vi "Connect.vi"(8 "error in (no error)":errorcluster, 10 "BaudRate":u32, 11 "VisaResource":string) -> (0 "error out":errorcluster, 3 "T560Session out":refnum<class "T560Session.lvclass">)   [LabVIEW 2020, in "Highland T564 DDG.lvclass"]
doc: "Connect to the physical device"
uses:
  Highland T564 DDG.lvclass
  T560Session.lvclass
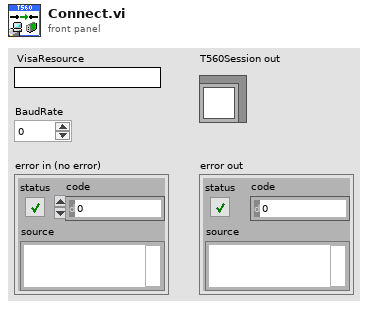
[diagram p1: front panel]
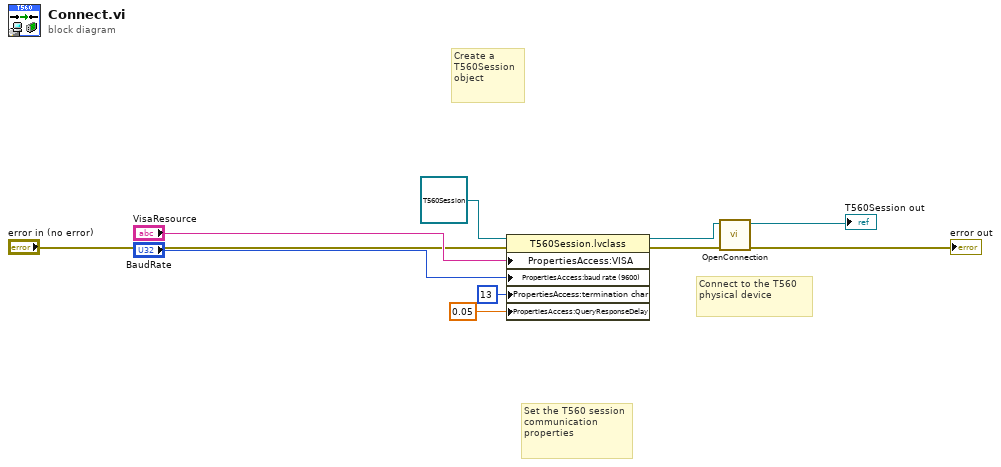
[diagram p0: block diagram]
diagram:
  # "Connect to the T560 physical device"
  # "Set the T560 session communication properties"
  # "Create a T560Session object"
  n1 = property class="T560Session.lvclass"(reference=refnum<class "T560Session.lvclass"> refnum ("Highlandt564.lvlib:T560Session.lvclass"), error in="error in (no error)", "PropertiesAccess:VISA"="VisaResource", "PropertiesAccess:baud rate (9600)"="BaudRate", "PropertiesAccess:termination char"=u8 13 ("termination char"), "PropertiesAccess:QueryResponseDelay"=0.05 ("QueryResponseDelay")) -> (reference out=w7:refnum<class "T560Session.lvclass">, error out=w6:errorcluster)
  n2 = call-dynamic "OpenConnection.vi"("error in"=w6, "T560Session in"=w7) -> ("error out"=→"error out":errorcluster, "T560Session out"=→"T560Session out":refnum<class "T560Session.lvclass">)  [unwired: 8 in]
